vi "Up and down1.vi"   [LabVIEW 2019]
uses:
  Supported.llb/Global-1.vi
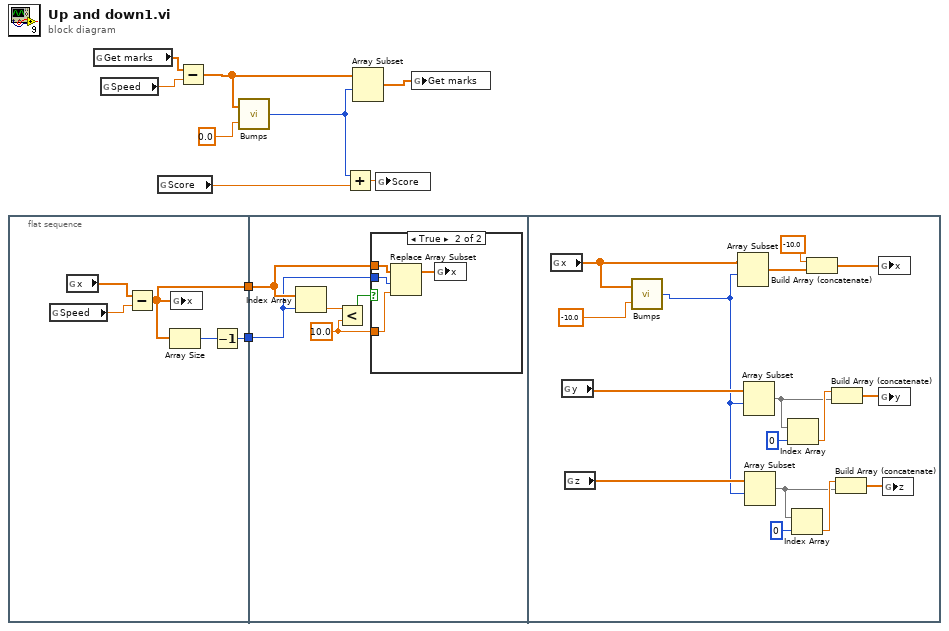
[diagram p0: block diagram]
diagram:
  n1 = flat-sequence {
    tunnel: [w11] -> w10
    tunnel: [w15] -> w9
    tunnel: w10 -> [w19]
    tunnel: w9 -> [w20]
    frame #0 {
      n2 = global read "Global-1.vi" "Speed"() -> (w13:dbl)
      n3 = global read "Global-1.vi" "x"() -> (w14:dbl[])
      n4 = Subtract(x=w14, y=w13) -> (x-y=w15:dbl[])
      n5 = Array Size(array=w15) -> (size(s)=w12:i32)
      n6 = global write "Global-1.vi" "x"(w15) -> ()
      n7 = Decrement(x=w12) -> (x-1=w11:i32)
    }
    frame #1 {
      w16 = 10.0 ("y")
      n8 = Index Array(array=w20, index=w19) -> (element=w18:dbl)
      n9 = Less?(x=w18, y=w16) -> (x < y?=w17:bool)
      n10 = case shown="True" w17 {
        tunnel: w20 -> [_ w24]
        tunnel: w19 -> [_ w22]
        tunnel: w16 -> [_ w21]
        frame False {
        }
        frame True {
          n11 = Replace Array Subset(array=w24, new element=w21, index=w22) -> (w23:dbl[])
          n12 = global write "Global-1.vi" "x"(w23) -> ()
        }
      }
    }
    frame #2 {
      n13 = global read "Global-1.vi" "x"() -> (w27:dbl[])
      n14 = global read "Global-1.vi" "y"() -> (w28:dbl[])
      n15 = global read "Global-1.vi" "z"() -> (w39:dbl[])
      n16 = call "Bumps.vi"("lower limit"=-10.0, "Array in"=w27) -> ("Index out"=w26:i32)
      n17 = Array Subset(array=w27, index=w26) -> (w38:dbl[])  [unwired: 1 in]
      n18 = Array Subset(array=w28, index=w26) -> (w35:dbl[])  [unwired: 1 in]
      n19 = Array Subset(array=w39, index=w26) -> (w30:dbl[])  [unwired: 1 in]
      n20 = Index Array(array=w35, index=0) -> (element=w36:dbl)
      n21 = Index Array(array=w30, index=0) -> (element=w32:dbl)
      n22 = Build Array (concatenate)(-10.0, w38) -> (w29:dbl[])
      n23 = Build Array (concatenate)(w36, w35) -> (w34:dbl[])
      n24 = Build Array (concatenate)(w32, w30) -> (w31:dbl[])
      n25 = global write "Global-1.vi" "x"(w29) -> ()
      n26 = global write "Global-1.vi" "y"(w34) -> ()
      n27 = global write "Global-1.vi" "z"(w31) -> ()
    }
  }
  n28 = global read "Global-1.vi" "Get marks"() -> (w4:dbl[])
  n29 = global read "Global-1.vi" "Speed"() -> (w5:dbl)
  n30 = global read "Global-1.vi" "Score"() -> (w6:dbl)
  n31 = Subtract(x=w4, y=w5) -> (x-y=w2:dbl[])
  n32 = call "Bumps.vi"("lower limit"=0.0, "Array in"=w2) -> ("Index out"=w1:i32)
  n33 = Add(x=w1, y=w6) -> (x+y=w7:dbl)
  n34 = Array Subset(array=w2, index=w1) -> (w8:dbl[])  [unwired: 1 in]
  n35 = global write "Global-1.vi" "Score"(w7) -> ()
  n36 = global write "Global-1.vi" "Get marks"(w8) -> ()
